vi "Vision Calculations.vi"() -> (3 "Joystick Values":dbl[](array[numeric]))   [LabVIEW 2017]
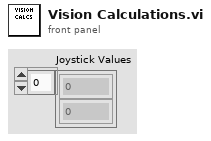
[diagram p1: front panel]
types:
  T1 = cluster{"Ratio Area":dbl, "Y":dbl, "X":dbl, "Total Area":dbl, "Timestamp":ext, "Height":dbl, "Width":dbl}
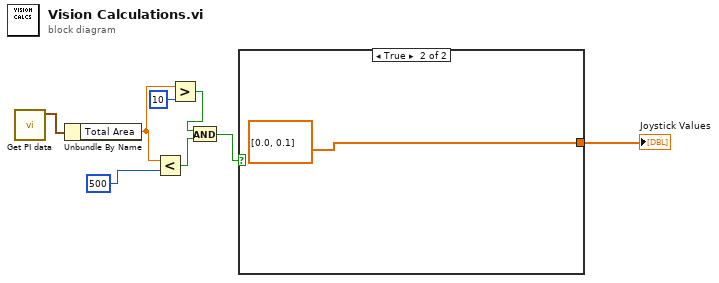
[diagram p0: block diagram]
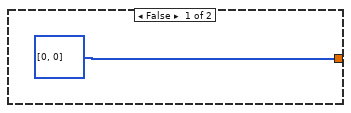
[diagram p2: hidden frame]
diagram:
  n1 = call "Get PI data.vi"() -> ("values"=w8:T1)  [unwired: 11 in]
  n2 = Unbundle By Name(w8) -> ("Total Area"=w5:dbl)
  n3 = Less?(x=w5, y=500) -> (x < y?=w2:bool)
  n4 = Greater?(x=w5, y=10) -> (0:w3:bool)
  n5 = And(x=w3, y=w2) -> (x .and. y?=w1:bool)
  n6 = case shown="True" w1 {
    tunnel: [i32[] [0, 0] dbl[] [0.0, 0.1]] -> w6
    frame False {
    }
    frame True {
    }
  }
  "Joystick Values" <- w6
